vi "Integer Field Formalise.vi"(8 "error in (no error)":errorcluster, 11 "Sudoku Class in":refnum<class "Sudoku Class.lvclass">) -> (0 "error out":errorcluster, 2 "Sudoku Formal":T1, 3 "Sudoku Class out":refnum<class "Sudoku Class.lvclass">)   [LabVIEW 2015, in "Sudoku Library.lvlib" / "Sudoku Class.lvclass"]
doc: "Created IvanLis by LabVIEW Portal\nProfile: http://labviewportal.org/memberlist.php?mode=viewprofile&u=987\neMail: IvanLisanov@gMail.com\nTelegram: https://t.me/IvanLis"
uses:
  Sudoku Class.lvclass
  TypeDef/Sudoku Formal.ctl
  TypeDef/Cell Formal.ctl
  Sudoku Class.lvclass/Sudoku Class.ctl
  Sudoku Library.lvlib
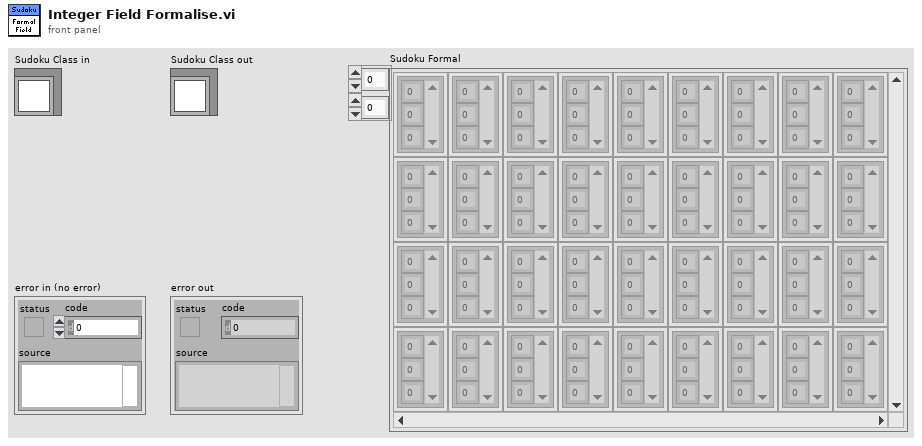
[diagram p1: front panel]
types:
  T1 = typedef "Sudoku Library.lvlib/Sudoku Formal.ctl" = T2[][]
  T2 = typedef "Sudoku Library.lvlib/Cell Formal.ctl" = cluster{"Variant":u8[]}
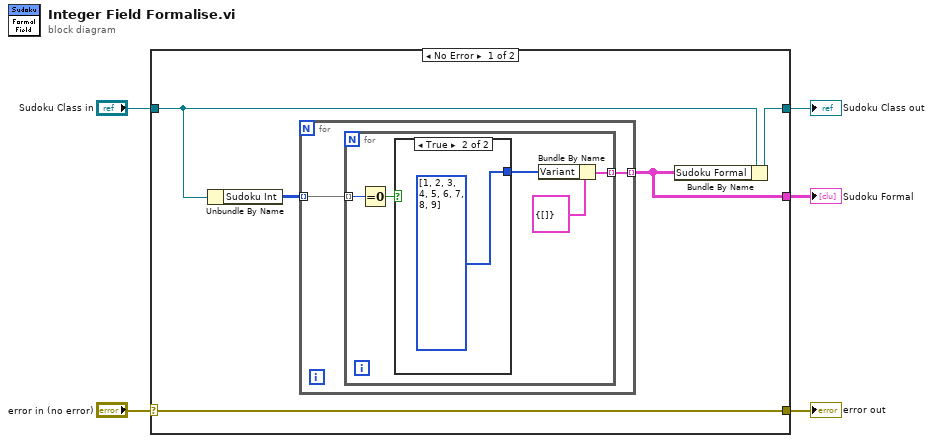
[diagram p0: block diagram]
diagram:
  n1 = case shown="No Error" "error in (no error)" {
    selector: "error in (no error)" -> [w10 w20]
    tunnel: [w10 w20] -> w4
    tunnel: [w8 w19] -> w2
    tunnel: "Sudoku Class in" -> [w9 w19]
    tunnel: [w6 _] -> w1
    frame No Error {
      n2 = Unbundle By Name(w9) -> ("Sudoku Int"=w7:u8[][])
      n3 = for {
        tunnel: w7 -> [w12] mode=indexing
        tunnel: [w11] -> w6 mode=indexing
        n4 = for {
          tunnel: w12 -> [w17] mode=indexing
          tunnel: [w14] -> w11 mode=indexing
          n5 = Equal To 0?(x=w17) -> (x = 0?=w16:bool)
          n6 = case shown="True" w16 {
            tunnel: [_ u8[] [1, 2, 3, 4, 5, 6, 7, 8, 9]] -> w13
            frame False {
            }
            frame True {
            }
          }
          n7 = Bundle By Name(cluster=T2 {"Variant"=[]} ("Cell"), "Variant"=w13) -> (w14:T2)
        }
      }
      n8 = Bundle By Name(cluster=w9, "Sudoku Formal"=w6) -> (w8:refnum<class "Sudoku Class.lvclass">)
    }
    frame Error {
    }
  }
  "error out" <- w4
  "Sudoku Class out" <- w2
  "Sudoku Formal" <- w1
